vi "MAP_FGV.vi"(8 "error in (no error)":errorcluster, 9 "DOs":bool[](array[boolean]), 11 "Relay_Channel_Out":T1[](array[typedef])) -> (0 "error out":errorcluster, 2 "DOs_out":bool[](array[boolean]), 3 "Relay_Channel_Out 2":T1[](array[typedef]))   [LabVIEW 2024, in "Relay_Module.lvlib"]
uses:
  Relay_Module.lvlib
  Relay_Enum_OUT.ctl
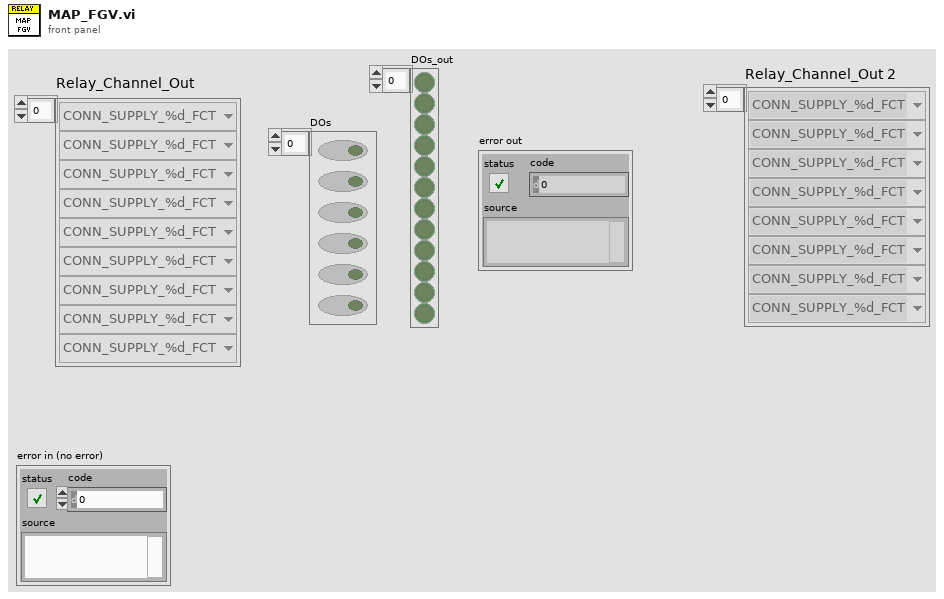
[diagram p1: front panel]
types:
  T1 = typedef "Relay_Module.lvlib/Relay_Enum_OUT.ctl" = enum16{"CONN_SUPPLY_%d_FCT", "HB_CONN_%d_FCT", "L_IND_CONN_%d_FCT", "R_IND_CONN_%d_FCT", "SW1_%d_FCT", "SW2_%d_FCT", "CAN_H_%d_FCT", "CAN_L_%d_FCT", "CYLINDER_ON/OFF_%d_FCT", "SPARE_1_%d_FCT", "SPARE_2_%d_FCT", "Tower Red", "Tower Amber", "Tower Green", "Tower Buzzer", "SLIMRELAY_DUT_%d_FCT", "GND_DMM_%d_EOL", "CAN_H_RES_%d_EOL", "CAN_L_RES_%d_EOL", "L_IND_RES_%d_EOL", "R_IND_RES_%d_EOL", "HB_CONN_DMM_%d_EOL", "14V_RES_%d_EOL", "CAN_L_(DMM-)_%d_EOL", "CAN_H_%d_EOL", "CAN_L_%d_EOL", "14V_%d_EOL", "GND_%d_EOL", "HB_CONN_%d_EOL", "L_IND_%d_EOL", "R_IND_%d_EOL", "CYLINDER_DUT_%d_EOL", "CYL_PB_1_%d_EOL", "CYL_PB_2_%d_EOL", "DUT_PASS_%d_EOL", "DUT_FAIL_%d_EOL", "SPARE1_%d_EOL", "Tower Red_EOL", "Tower Amber_EOL", "Tower Green_EOL", "Tower Buzzer_EOL"}
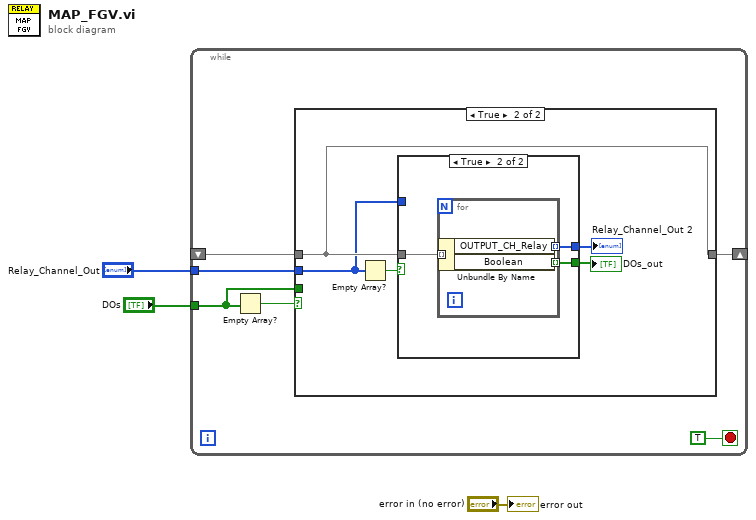
[diagram p0: block diagram]
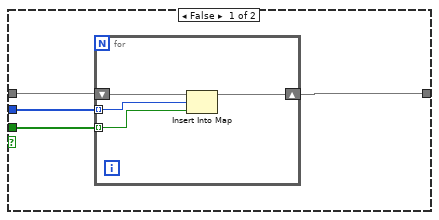
[diagram p2: hidden frame]
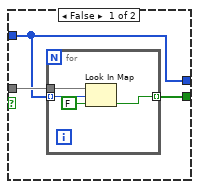
[diagram p3: hidden frame]
diagram:
  n1 = while {
    tunnel: "DOs" -> [w6]
    tunnel: "Relay_Channel_Out" -> [w7]
    shift-right: [w5] -> _
    shift-left: _ -> [w4]
    stop <- TRUE stop-if-true
    n2 = Empty Array?(array=w6) -> (empty?=w8:bool)
    n3 = case shown="True" w8 {
      tunnel: w7 -> [w13 w20]
      tunnel: w6 -> [w12 _]
      tunnel: [w11 w21] -> w5
      tunnel: w4 -> [w10 w21]
      frame False {
        n4 = for {
          tunnel: w13 -> [w17] mode=indexing
          tunnel: w12 -> [w16] mode=indexing
          shift-right: [w15] -> w11
          shift-left: w10 -> [w14]
          n5 = Insert Into Map(map in=w14, key=w17, value=w16) -> (map out=w15:map{T1, bool})  [unwired: 2 out]
        }
      }
      frame True {
        n6 = Empty Array?(array=w20) -> (empty?=w22:bool)
        n7 = case shown="True" w22 {
          tunnel: w21 -> [w25 w32]
          tunnel: [w23 w30] -> w18
          tunnel: [w24 w31] -> w19
          tunnel: w20 -> [w23 _]
          frame False {
            n8 = for {
              tunnel: w25 -> [w29]
              tunnel: [w28] -> w24 mode=indexing
              tunnel: w23 -> [w27] mode=indexing
              n9 = Look In Map(map=w29, key=w27, default value=FALSE) -> (value=w28:bool)  [unwired: 1 out]
            }
          }
          frame True {
            n10 = for {
              tunnel: w32 -> [w35] mode=indexing
              tunnel: [w34] -> w30 mode=indexing
              tunnel: [w33] -> w31 mode=indexing
              n11 = Unbundle By Name(w35) -> ("OUTPUT_CH_Relay"=w34:T1, "Boolean"=w33:bool)
            }
          }
        }
        "DOs_out" <- w19
        "Relay_Channel_Out 2" <- w18
      }
    }
  }
  "error out" <- "error in (no error)"
